vi "初始化.vi"(8 "error in (no error)":errorcluster caption="错误输入（无错误）", 9 "数据":T1, 11 "程序响应 输入":refnum<class "程序响应.lvclass">) -> (0 "error out":errorcluster caption="错误输出", 3 "程序响应 输出":refnum<class "程序响应.lvclass">)   [LabVIEW 2020, in "程序响应.lvlib" / "程序响应.lvclass"]
uses:
  D:/SuperPython-master/AutocompleteMenu-ScintillaNET.dll
  AutocompleteMenu-ScintillaNET.dll
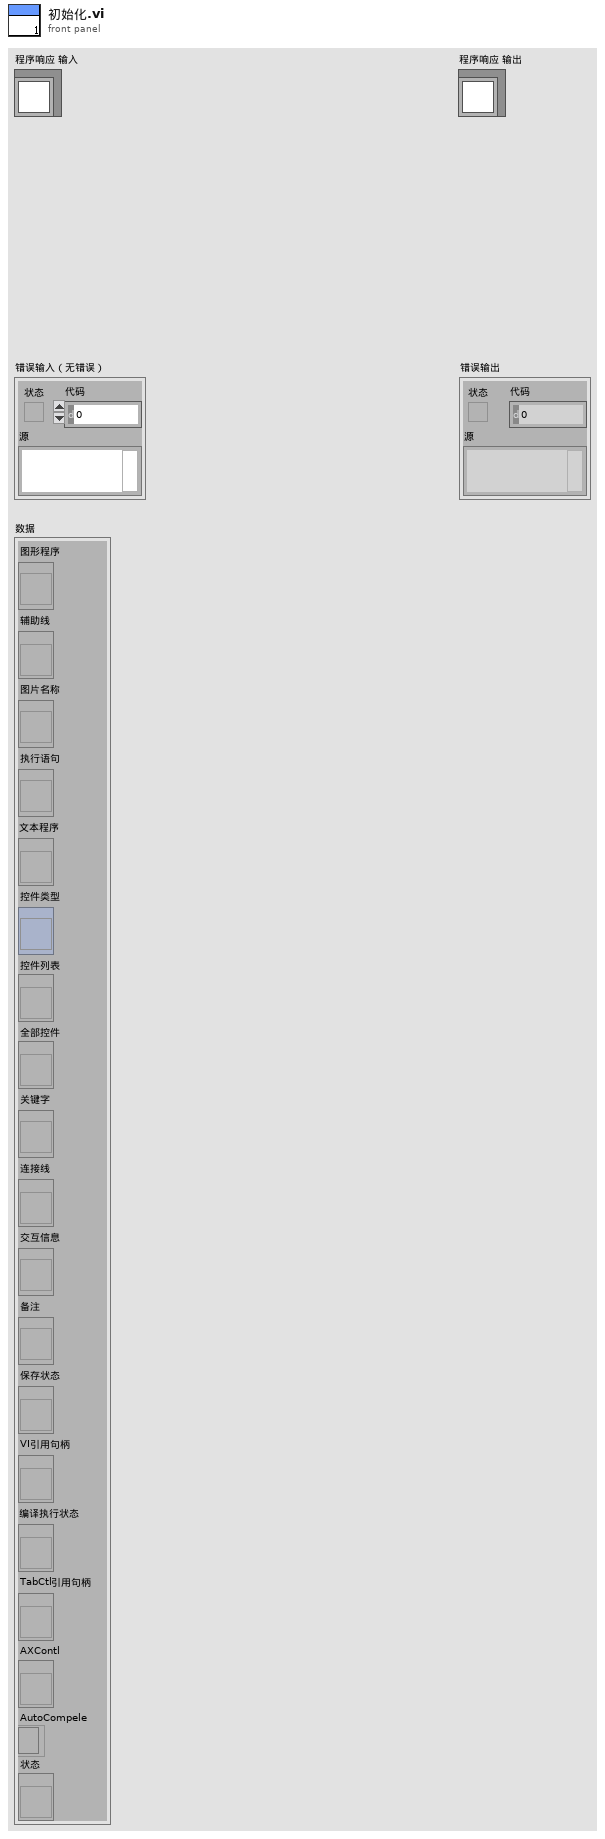
[diagram p1: front panel]
types:
  T1 = cluster{"图形程序":refnum<vi>, "辅助线":refnum<vi>, "图片名称":refnum<vi>, "执行语句":refnum<vi>, "文本程序":refnum<vi>, "控件类型":refnum<vi>, "控件列表":refnum<vi>, "全部控件":refnum<vi>, "关键字":refnum<vi>, "连接线":refnum<vi>, "交互信息":refnum<vi>, "备注":refnum<vi>, "保存状态":refnum<vi>, "VI引用句柄":refnum<vi>, "编译执行状态":refnum<vi>, "TabCtl引用句柄":refnum<vi>, "AXContl":refnum<vi>, "AutoCompele":refnum<k24>, "状态":refnum<vi>}
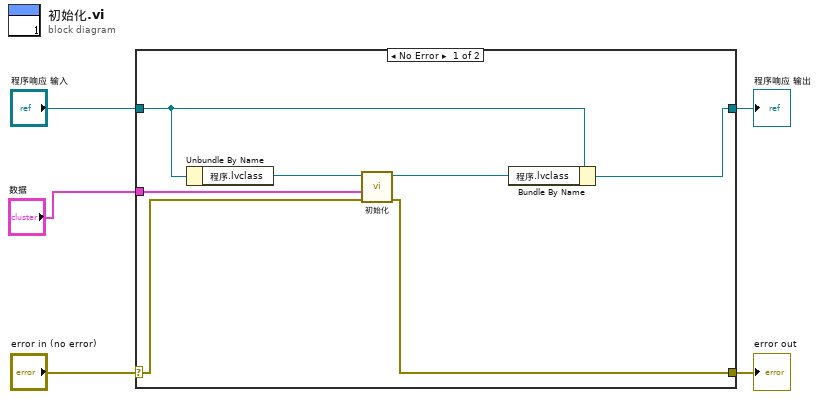
[diagram p0: block diagram]
diagram:
  n1 = case shown="No Error" "error in (no error)" {
    selector: "error in (no error)" -> [w7 w14]
    tunnel: [w6 w14] -> w4
    tunnel: [w9 w13] -> w2
    tunnel: "程序响应 输入" -> [w11 w13]
    tunnel: "数据" -> [w8 _]
    frame No Error {
      n2 = Unbundle By Name(w11) -> ("程序.lvclass"=w12:refnum<class "程序.lvclass">)
      n3 = call-dynamic "初始化.vi"("error in (no error)"=w7, "数据"=w8, "程序 输入"=w12) -> ("error out"=w6:errorcluster, "程序 输出"=w10:refnum<class "程序.lvclass">)  [unwired: 7 in]
      n4 = Bundle By Name(cluster=w11, "程序.lvclass"=w10) -> (w9:refnum<class "程序响应.lvclass">)
    }
    frame Error {
    }
  }
  "error out" <- w4
  "程序响应 输出" <- w2
